vi "main-log-viewer.vi"() -> ()   [LabVIEW 2016]
uses:
  <vilib>/addons/h5labview2/base/lib_path.vi
  <vilib>/addons/h5labview2/base/H5Equery.vi
  <vilib>/addons/h5labview2/dataset/H5Dread.llb/H5Dread.xnode
  <vilib>/addons/h5labview2/file/H5F.lvlib
panel:
  out "XY Graph":cluster{timestamp[], sgl[]}[](graph)
  in  "stop":bool
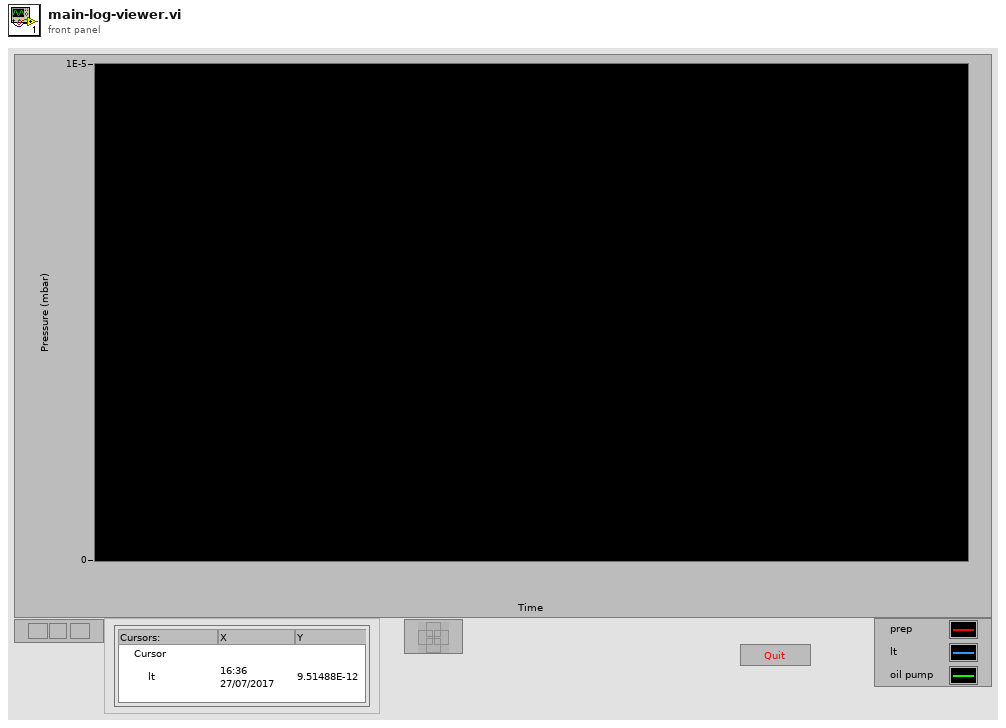
[diagram p1: front panel]
types:
  T1 = cluster{"timestamp":i64, "time <19>":string, "prep":sgl, "lt":sgl, "prevacuum":sgl}
  T2 = typedef "hid_t.ctl" = i32
  T3 = cluster{"timestamp":i64, "time <19>":string, "prep":sgl, "lt":sgl, "prevacuum":sgl}[]
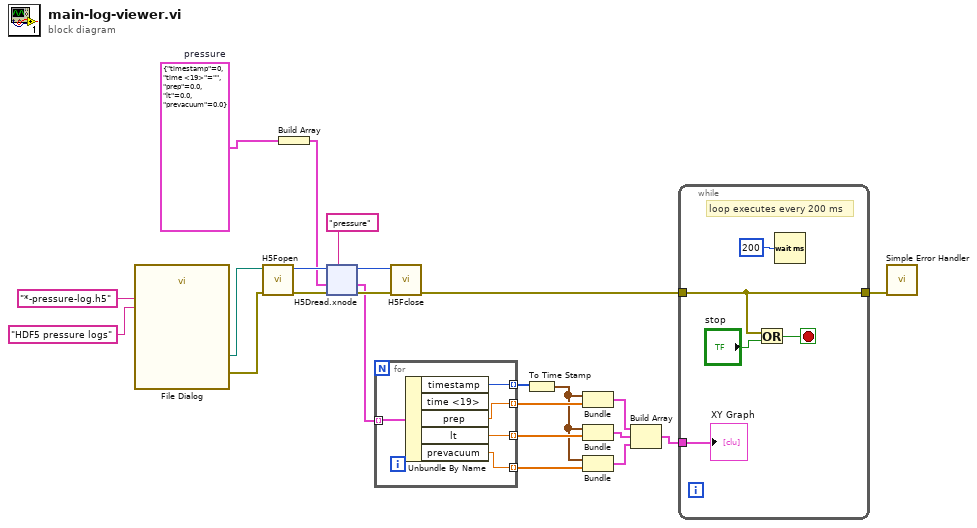
[diagram p0: block diagram]
diagram:
  w15 = T1 {"timestamp"=0, "time <19>"="", "prep"=0.0, "lt"=0.0, "prevacuum"=0.0}  # pressure
  n1 = call "File Dialog"("pattern (all files)"="*-pressure-log.h5", "pattern label"="HDF5 pressure logs") -> ("selected path"=w23:path, "error out"=w19:errorcluster)  [unwired: 10 in, 2 out]
  n2 = call <vilib>:"H5Fopen.vi"("error in (no error)"=w19, "path"=w23) -> ("error out"=w20:errorcluster, "ref out"=w22:T2)  [unwired: 8 in]
  n3 = Build Array(w15) -> (w14:T3)
  n4 = xnode "H5Dread.xnode"("dataset name (this)"="pressure", "error in (no error)"=w20, "default"=w14, "ref in"=w22) -> ("error out"=w18:errorcluster, "data"=w12:T3, "ref out"=w21:i32)  [unwired: 2 in, 1 out]
  n5 = for {
    tunnel: w12 -> [w28] mode=indexing
    tunnel: [w27] -> w6 mode=indexing
    tunnel: [w26] -> w11 mode=indexing
    tunnel: [w25] -> w8 mode=indexing
    tunnel: [w24] -> w7 mode=indexing
    n6 = Unbundle By Name(w28) -> ("timestamp"=w27:i64, "prep"=w26:sgl, "lt"=w25:sgl, "prevacuum"=w24:sgl)  [unwired: 1 out]
  }
  n7 = call <vilib>:"H5Fclose.vi"("error in (no error)"=w18, "ref"=w21) -> ("error out"=w10:errorcluster)  [unwired: 9 in]
  n8 = To Time Stamp(1:w6) -> (0:w1:timestamp[])
  n9 = Bundle(w1, w11) -> (w5:cluster{timestamp[], sgl[]})  [unwired: 1 in]
  n10 = Bundle(w1, w8) -> (w4:cluster{timestamp[], sgl[]})  [unwired: 1 in]
  n11 = Bundle(w1, w7) -> (w3:cluster{timestamp[], sgl[]})  [unwired: 1 in]
  n12 = Build Array(w5, w4, w3) -> (w2:cluster{timestamp[], sgl[]}[])
  n13 = while {
    tunnel: w10 -> [w29]
    tunnel: [w29] -> w9
    tunnel: w2 -> [w32]
    stop <- w33 stop-if-true
    # "loop executes every 200 ms"
    n14 = Or(x=w29, y="stop") -> (x .or. y?=w33:bool)
    n15 = Wait (ms)(milliseconds to wait=u32 200) -> ()  [unwired: 1 out]
    "XY Graph" <- w32
  }
  n16 = call <vilib>:"Simple Error Handler.vi"("error in (no error)"=w9) -> ()  [unwired: 4 in, 5 out]
